vi "FTW-Logger-FlushToFile.vi"(0 "FTW Logger":refnum<class "FTW-Logger-Core.lvclass">, 11 "error in":errorcluster) -> (4 "FTW Logger out":refnum<class "FTW-Logger-Core.lvclass">, 15 "error out":errorcluster)   [LabVIEW 2013, in "FTW-Actor.lvlib" / "FTW-Logger-Core.lvclass"]
uses:
  FTW-Logger-Core.lvclass
  FTW-Logger-Core.lvclass/FTW-Logger-Core.ctl
panel:
  # "Inputs"
  # "Outputs"
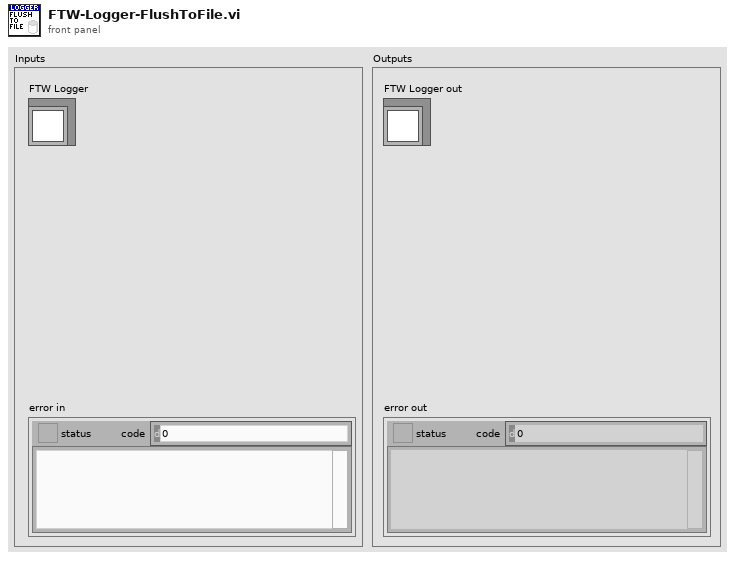
[diagram p1: front panel]
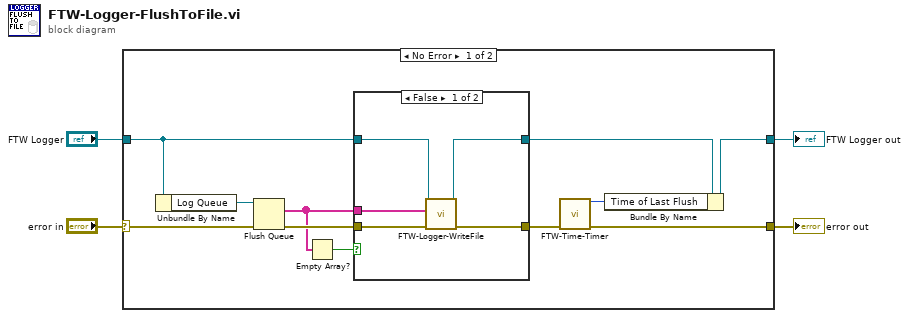
[diagram p0: block diagram]
diagram:
  n1 = case shown="No Error" "error in" {
    selector: "error in" -> [w9 w24]
    tunnel: [w8 w24] -> w1
    tunnel: [w6 w23] -> w3
    tunnel: "FTW Logger" -> [w10 w23]
    frame No Error {
      n2 = Unbundle By Name(w10) -> ("Log Queue"=w15:refnum<queue>)
      n3 = Flush Queue(queue=w15, error in (no error)=w9) -> (remaining elements=w13:string[], error out=w14:errorcluster)  [unwired: 1 out]
      n4 = Empty Array?(array=w13) -> (empty?=w12:bool)
      n5 = case shown="False" w12 {
        tunnel: [w20 w21] -> w7
        tunnel: w14 -> [w19 w21]
        tunnel: w13 -> [w18 _]
        tunnel: w10 -> [w17 w22]
        tunnel: [w16 w22] -> w11
        frame False {
          n6 = call "FTW-Logger-WriteFile.vi"("FTW Logger"=w17, "Entries to Log"=w18, "error in"=w19) -> ("FTW Logger out"=w16:refnum<class "FTW-Logger-Core.lvclass">, "error out"=w20:errorcluster)  [unwired: 11 in]
        }
        frame True {
        }
      }
      n7 = call "FTW-Time-Timer.vi"("error in"=w7) -> ("Current Tick Count"=w5:u32, "error out"=w8:errorcluster)  [unwired: 12 in, 1 out]
      n8 = Bundle By Name(cluster=w11, "Time of Last Flush"=w5) -> (w6:refnum<class "FTW-Logger-Core.lvclass">)
    }
    frame Error {
    }
  }
  "error out" <- w1
  "FTW Logger out" <- w3
